vi "addFailure.vi"(7 "execution time (sec)":dbl, 8 "error in (no error)":errorcluster, 9 "test error":errorcluster, 10 "test":refnum<class>, 11 "TestTestResult in":refnum<class "_TextTestResult.lvclass">) -> (0 "error out":errorcluster, 3 "TestTestResult out":refnum<class "_TextTestResult.lvclass">)   [LabVIEW 2011, in "_TextTestResult.lvclass"]
uses:
  _TextTestResult.lvclass
  TestCase/TestCase.lvclass
  TestResult/TestResult.lvclass
  _TextTestResult.lvclass/_TextTestResult.ctl
panel:
  # "JKI VI Tester for LabVIEW\nhttp://jkisoft.com/vi-tester\nCopyright (C) 2007-2009, JKI <info@jkisoft.com>\nALL RIGHTS RESERVED"
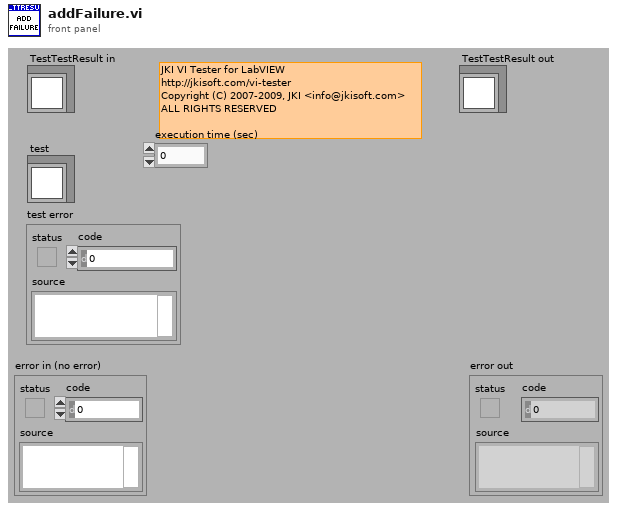
[diagram p1: front panel]
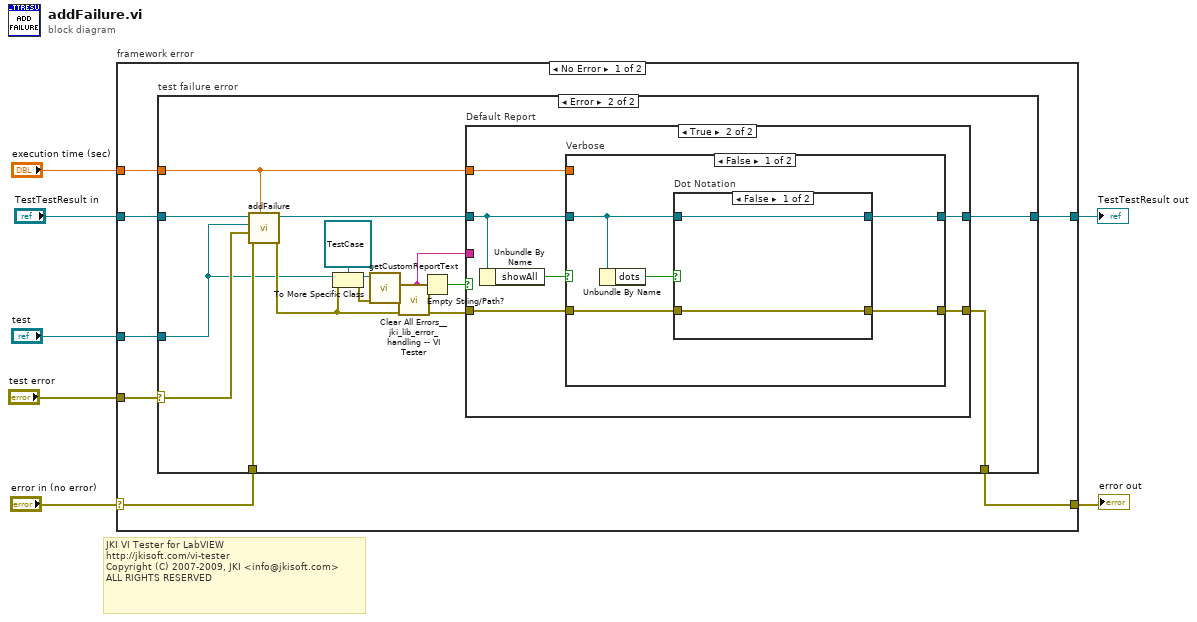
[diagram p0: block diagram]
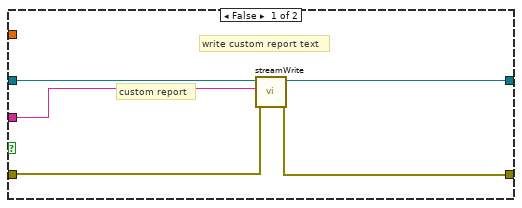
[diagram p3: hidden frame]
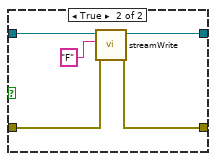
[diagram p4: hidden frame]
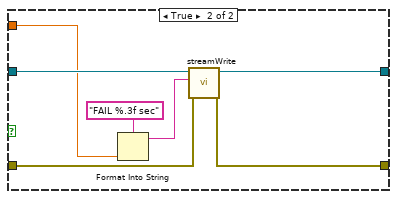
[diagram p5: hidden frame]
diagram:
  # "JKI VI Tester for LabVIEW\nhttp://jkisoft.com/vi-tester\nCopyright (C) 2007-2009, JKI <info@jkisoft.com>\nALL RIGHTS RESERVED"
  n1 = case "framework error" shown="No Error" "error in (no error)" {
    selector: "error in (no error)" -> [w12 w63]
    tunnel: [w11 w63] -> w6
    tunnel: [w13 w62] -> w4
    tunnel: "TestTestResult in" -> [w14 w62]
    tunnel: "test" -> [w10 _]
    tunnel: "test error" -> [w9 _]
    tunnel: "execution time (sec)" -> [w8 _]
    frame No Error {
      n2 = case "test failure error" shown="Error" w9 {
        selector: w9 -> [_ w26]
        tunnel: w14 -> [w16 w30]
        tunnel: [w16 w29] -> w13
        tunnel: w12 -> [w15 w28]
        tunnel: [w15 w27] -> w11
        tunnel: w10 -> [_ w17]
        tunnel: w8 -> [_ w25]
        frame No Error {
        }
        frame Error {
          n3 = call-parent "addFailure.vi"("execution time (sec)"=w25, "error in (no error)"=w28, "test error"=w26, "test"=w17, "TestResult in"=w30) -> ("error out"=w20:errorcluster, "TestResult out"=w31:refnum<class "_TextTestResult.lvclass">)  [unwired: 5 in]
          n4 = To More Specific Class(target class=refnum<class "TestCase.lvclass"> refnum ("TestCase in"), reference=w17, error in=w20) -> (specific class reference=w22:refnum<class "TestCase.lvclass">, error out=w24:errorcluster)
          n5 = call-dynamic "getCustomReportText.vi"("error in (no error)"=w24, "TestCase in"=w22) -> ("error out"=w21:errorcluster, "customReportText"=w18:string)  [unwired: 7 in, 1 out]
          n6 = call "Clear All Errors__jki_lib_error_handling -- VI Tester.vi"("error in"=w21) -> ()  [unwired: 4 in, 1 out]
          n7 = Empty String/Path?(string/path=w18) -> (empty?=w19:bool)
          n8 = case "Default Report" shown="True" w19 {
            tunnel: w31 -> [w36 w41]
            tunnel: [w32 w40] -> w29
            tunnel: [w33 w39] -> w27
            tunnel: w25 -> [_ w38]
            tunnel: w20 -> [w34 w37]
            tunnel: w18 -> [w35 _]
            frame False {
              # "custom report"
              # "write custom report text"
              n9 = call "streamWrite.vi"("error in (no error)"=w34, "String"=w35, "TestTestResult in"=w36) -> ("error out"=w33:errorcluster, "TestTestResult out"=w32:refnum<class "_TextTestResult.lvclass">)  [unwired: 7 in]
            }
            frame True {
              n10 = Unbundle By Name(w41) -> ("showAll"=w42:bool)
              n11 = case "Verbose" shown="False" w42 {
                tunnel: w41 -> [w46 w61]
                tunnel: w37 -> [w44 w59]
                tunnel: [w43 w58] -> w39
                tunnel: [w47 w60] -> w40
                tunnel: w38 -> [_ w57]
                frame False {
                  n12 = Unbundle By Name(w46) -> ("dots"=w45:bool)
                  n13 = case "Dot Notation" shown="False" w45 {
                    tunnel: w46 -> [w48 w54]
                    tunnel: w44 -> [w49 w51]
                    tunnel: [w49 w50] -> w43
                    tunnel: [w48 w53] -> w47
                    frame False {
                    }
                    frame True {
                      n14 = call "streamWrite.vi"("error in (no error)"=w51, "String"="F" ("element"), "TestTestResult in"=w54) -> ("error out"=w50:errorcluster, "TestTestResult out"=w53:refnum<class "_TextTestResult.lvclass">)  [unwired: 7 in]
                    }
                  }
                }
                frame True {
                  n15 = Format Into String(format string="FAIL %.3f sec" ("element"), w57) -> (resulting string=w55:string)  [unwired: 2 in, 1 out]
                  n16 = call "streamWrite.vi"("error in (no error)"=w59, "String"=w55, "TestTestResult in"=w61) -> ("error out"=w58:errorcluster, "TestTestResult out"=w60:refnum<class "_TextTestResult.lvclass">)  [unwired: 7 in]
                }
              }
            }
          }
        }
      }
    }
    frame Error {
    }
  }
  "error out" <- w6
  "TestTestResult out" <- w4
